vi "Read Pitch Roll Yaw.vi"(8 "error in":errorcluster, 11 "Orient3d Class in":refnum<class "Orient3d Class.lvclass">) -> (0 "error out":errorcluster, 1 "yaw":dbl, 2 "roll":dbl, 3 "pitch":dbl)   [LabVIEW 2011, in "Orient3d Class.lvclass"]
uses:
  Orient3d Class.lvclass
  Orient3d Class.lvclass/Orient3d Class.ctl
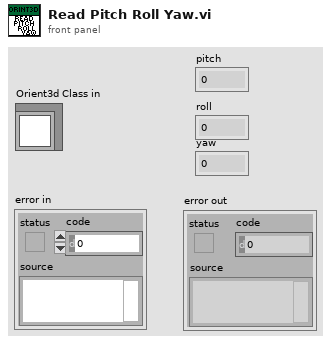
[diagram p1: front panel]
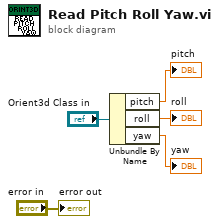
[diagram p0: block diagram]
diagram:
  n1 = Unbundle By Name("Orient3d Class in") -> ("pitch"=→"pitch":dbl, "roll"=→"roll":dbl, "yaw"=→"yaw":dbl)
  "error out" <- "error in"
